vi "MICSD Search for Implant.vi"(0 "VISA Resource Name":refnum<visa-resource-name>, 1 "Search Time (mS)":u32=3000, 5 "Enable Watchdog?(T)":bool=TRUE, 7 "Any Company?(T)":bool=TRUE, 9 "Any Implant?(T)":bool=TRUE, 11 "error in (no error)":errorcluster) -> (4 "dup VISA Resource Name":refnum<visa-resource-name>, 6 "Device Found?":bool, 8 "Detected MICS IDs":u32[](array[numeric]) format="%06x", 15 "error out":errorcluster)   [LabVIEW 2020]
uses:
  <vilib>/Instr/_visa.llb/VISA Configure Serial Port (Instr).vi
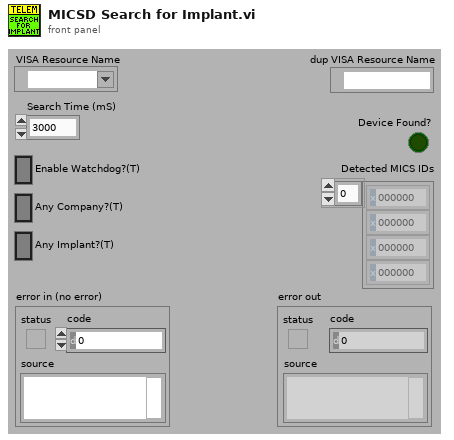
[diagram p1: front panel]
types:
  T1 = cluster{"Command Token":u8, "Length":u16, "Pack Data":u8[]}
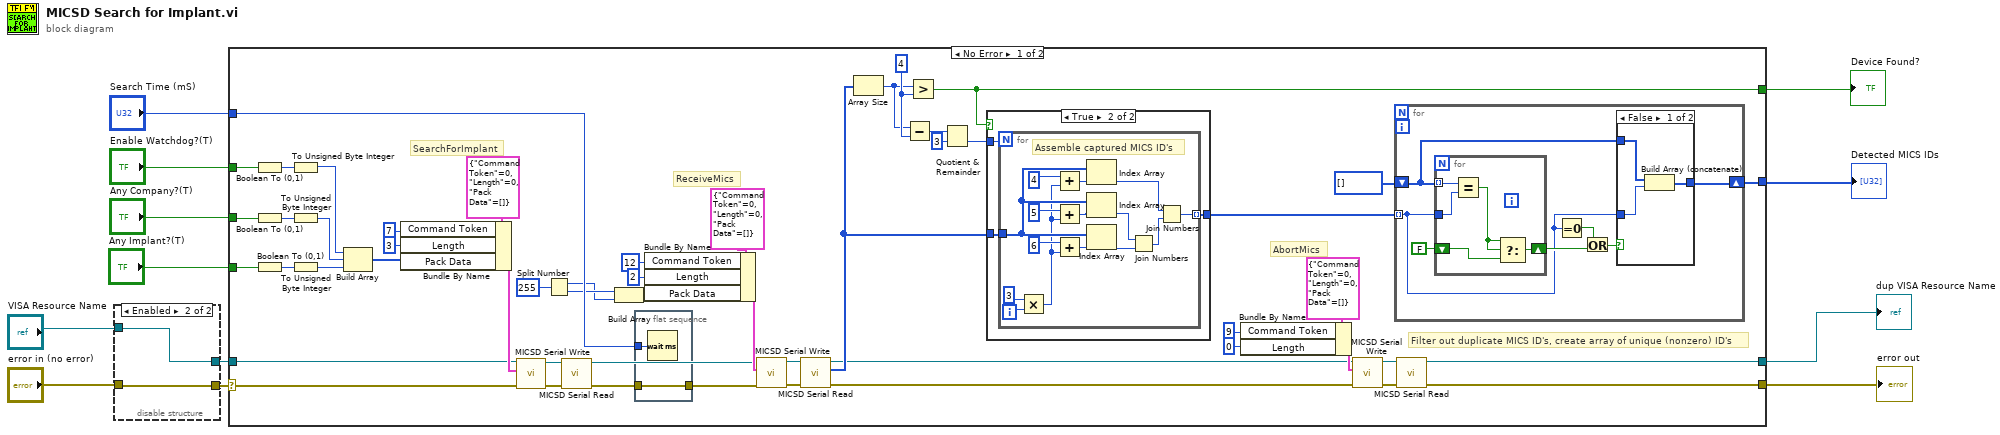
[diagram p0: block diagram]
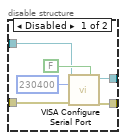
[diagram p2: hidden frame]
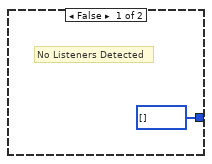
[diagram p4: hidden frame]
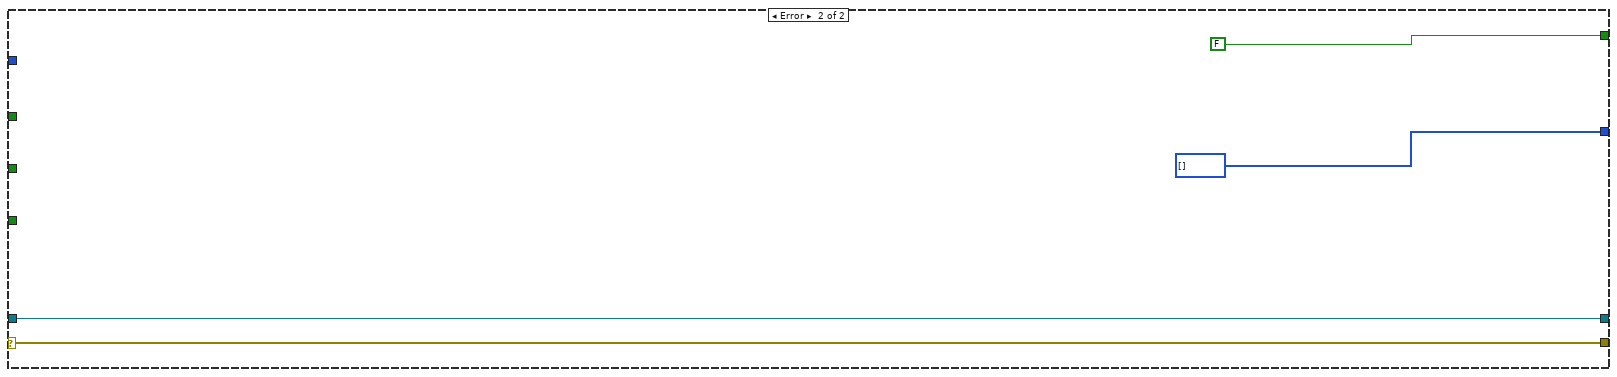
[diagram p5: hidden frame]
diagram:
  n1 = disable-structure shown="Enabled" {
    disable-tunnel: [w16 w19] -> w6
    disable-tunnel: [w15 w20] -> w5
    disable-tunnel: "VISA Resource Name" -> [w14 w20]
    disable-tunnel: "error in (no error)" -> [w13 w19]
    frame Disabled {
      n2 = call-poly "VISA Configure Serial Port"("VISA resource name"=w14, "Enable Termination\nChar (T)"=FALSE ("Enable Termination\nChar (T)"), "baud rate (9600)"=u32 230400, "error in (no error)"=w13) -> ("VISA resource name out"=w15:refnum<visa-resource-name>, "error out"=w16:errorcluster)  [unwired: 10 in]
    }
    frame Enabled {
    }
  }
  n3 = case shown="No Error" w6 {
    selector: w6 -> [w67 w110]
    tunnel: w5 -> [w68 w111]
    tunnel: "Enable Watchdog?(T)" -> [w66 _]
    tunnel: "Any Company?(T)" -> [w65 _]
    tunnel: "Any Implant?(T)" -> [w64 _]
    tunnel: "Search Time (mS)" -> [w55 _]
    tunnel: [w41 w110] -> w1
    tunnel: [w40 w111] -> w2
    tunnel: [w49 FALSE] -> w8
    tunnel: [w21 u32[] []] -> w7
    frame No Error {
      w26 = u16 4 ("Length")
      # "Filter out duplicate MICS ID's, create array of unique (nonzero) ID's"
      # "AbortMics"
      # "ReceiveMics"
      # "SearchForImplant"
      n4 = Boolean To (0,1)(Boolean=w66) -> (0, 1=w63:i16)
      n5 = Boolean To (0,1)(Boolean=w65) -> (0, 1=w62:i16)
      n6 = Boolean To (0,1)(Boolean=w64) -> (0, 1=w61:i16)
      n7 = To Unsigned Byte Integer(number=w63) -> (unsigned 8bit integer=w60:u8)
      n8 = To Unsigned Byte Integer(number=w62) -> (unsigned 8bit integer=w59:u8)
      n9 = To Unsigned Byte Integer(number=w61) -> (unsigned 8bit integer=w58:u8)
      n10 = Build Array(w60, w59, w58) -> (w57:u8[])
      n11 = Bundle By Name(cluster=T1 {"Command Token"=0, "Length"=0, "Pack Data"=[]} ("Write Data"), "Command Token"=u8 7, "Length"=u16 3, "Pack Data"=w57) -> (w72:T1)
      n12 = call "MICSD Serial Write.vi"("error in (no error)"=w67, "Write Data"=w72, "VISA Resource Name"=w68) -> ("error out"=w27:errorcluster, "DUP Visa Resource Name"=w29:refnum<visa-resource-name>)  [unwired: 7 in]
      n13 = Split Number(x=u16 255 ("Command Token")) -> (hi(x)=w35:u8, lo(x)=w36:u8)
      n14 = call "MICSD Serial Read.vi"("error in (no error)"=w27, "VISA Resource Name"=w29) -> ("error out"=w56:errorcluster, "DUP Visa Resource Name"=w45:refnum<visa-resource-name>)  [unwired: 7 in, 1 out]
      n15 = Build Array(w36, w35) -> (w50:u8[])
      n16 = flat-sequence {
        tunnel: w56 -> [w109]
        tunnel: [w109] -> w28
        tunnel: w55 -> [w108]
        frame #0 {
          n17 = Wait (ms)(milliseconds to wait=w108) -> ()  [unwired: 1 out]
        }
      }
      n18 = Bundle By Name(cluster=T1 {"Command Token"=0, "Length"=0, "Pack Data"=[]} ("Write Data"), "Command Token"=u8 12, "Length"=u16 2, "Pack Data"=w50) -> (w54:T1)
      n19 = call "MICSD Serial Write.vi"("error in (no error)"=w28, "Write Data"=w54, "VISA Resource Name"=w45) -> ("error out"=w33:errorcluster, "DUP Visa Resource Name"=w32:refnum<visa-resource-name>)  [unwired: 7 in]
      n20 = call "MICSD Serial Read.vi"("error in (no error)"=w33, "VISA Resource Name"=w32) -> ("error out"=w39:errorcluster, "Read Data"=w46:u8[], "DUP Visa Resource Name"=w37:refnum<visa-resource-name>)  [unwired: 7 in]
      n21 = Array Size(array=w46) -> (size(s)=w25:i32)
      n22 = Subtract(x=w25, y=w26) -> (x-y=w24:i32)
      n23 = Greater?(x=w25, y=w26) -> (0:w49:bool)
      n24 = Quotient & Remainder(x=w24, y=u16 3 ("Length")) -> (floor(x/y)=w48:i32)  [unwired: 1 out]
      n25 = case shown="True" w49 {
        tunnel: w48 -> [_ w92]
        tunnel: w46 -> [_ w91]
        tunnel: [u32[] [] w90] -> w23
        frame False {
          # "No Listeners Detected"
        }
        frame True {
          n26 = for {
            N: w92 -> [_]
            tunnel: w91 -> [w105]
            tunnel: [w100] -> w90 mode=indexing
            i -> [w107]
            # "Assemble captured MICS ID's"
            n27 = Multiply(x=u16 3 ("Length"), y=w107) -> (x*y=w96:i32)
            n28 = Add(x=u16 4 ("Length"), y=w96) -> (x+y=w95:i32)
            n29 = Add(x=u16 5 ("Length"), y=w96) -> (x+y=w94:i32)
            n30 = Add(x=u16 6 ("Length"), y=w96) -> (x+y=w93:i32)
            n31 = Index Array(array=w105, index=w95) -> (element=w101:u8)
            n32 = Index Array(array=w105, index=w94) -> (element=w103:u8)
            n33 = Index Array(array=w105, index=w93) -> (element=w104:u8)
            n34 = Join Numbers(hi=w103, lo=w104) -> ((hi.lo)=w102:u16)
            n35 = Join Numbers(hi=w101, lo=w102) -> ((hi.lo)=w100:u32)
          }
        }
      }
      n36 = Bundle By Name(cluster=T1 {"Command Token"=0, "Length"=0, "Pack Data"=[]} ("Write Data"), "Command Token"=u8 9, "Length"=u16 0) -> (w44:T1)
      n37 = call "MICSD Serial Write.vi"("error in (no error)"=w39, "Write Data"=w44, "VISA Resource Name"=w37) -> ("error out"=w30:errorcluster, "DUP Visa Resource Name"=w31:refnum<visa-resource-name>)  [unwired: 7 in]
      n38 = for {
        tunnel: w23 -> [w73] mode=indexing
        shift-right: [w78] -> w21
        shift-left: u32[] [] -> [w77]
        n39 = for {
          tunnel: w77 -> [w88] mode=indexing
          tunnel: w73 -> [w85]
          shift-right: [w87] -> w76
          shift-left: FALSE -> [w86]
          n40 = Equal?(x=w88, y=w85) -> (x = y?=w84:bool)
          n41 = Select(t=w84, s=w84, f=w86) -> (s? t:f=w87:bool)
        }
        n42 = Equal To 0?(x=w73) -> (x = 0?=w74:bool)
        n43 = Or(x=w74, y=w76) -> (x .or. y?=w75:bool)
        n44 = case shown="False" w75 {
          tunnel: w73 -> [w82 _]
          tunnel: [w81 w83] -> w78
          tunnel: w77 -> [w80 w83]
          frame False {
            n45 = Build Array (concatenate)(w80, w82) -> (w81:u32[])
          }
          frame True {
          }
        }
      }
      n46 = call "MICSD Serial Read.vi"("error in (no error)"=w30, "VISA Resource Name"=w31) -> ("error out"=w41:errorcluster, "DUP Visa Resource Name"=w40:refnum<visa-resource-name>)  [unwired: 7 in, 1 out]
    }
    frame Error {
    }
  }
  "Detected MICS IDs" <- w7
  "dup VISA Resource Name" <- w2
  "error out" <- w1
  "Device Found?" <- w8
